vi "TC Max and Min Benchmark.vi"() -> ()   [LabVIEW 2010]
uses:
  <vilib>/eio/EIONode/EIONode.xnode
panel:
  out "Minimum Reached":fxp<+/-,24,-2> format="%.26g"
  out "Maximum Reached":fxp<+/-,24,-2> format="%.26g"
  out "Current TC Signal":fxp<+/-,24,-2> format="%.26g"
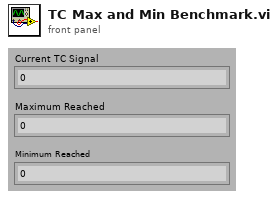
[diagram p1: front panel]
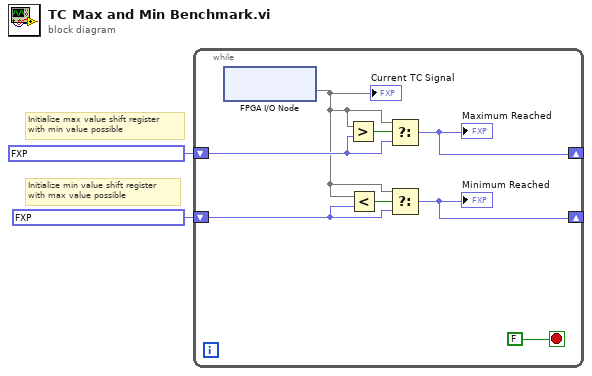
[diagram p0: block diagram]
diagram:
  # "Initialize max value shift register\nwith min value possible"
  # "Initialize min value shift register\nwith max value possible"
  n1 = while {
    shift-right: [w7] -> _
    shift-left: fxp<+/-,24,-2> -0.125 -> [w8]
    shift-right: [w3] -> _
    shift-left: fxp<+/-,24,-2> 0.1249999850988388 -> [w4]
    stop <- FALSE stop-if-true
    n2 = xnode "FPGA I/O Node"() -> ("Mod1/TC0"=w5)  [unwired: 1 in, 1 out]
    "Current TC Signal" <- w5
    n3 = Greater?(x=w5, y=w8) -> (0:w9:bool)
    n4 = Less?(x=w5, y=w4) -> (x < y?=w6:bool)
    n5 = Select(t=w5, s=w9, f=w8) -> (s? t:f=w7:fxp<+/-,24,-2>)
    "Maximum Reached" <- w7
    n6 = Select(t=w5, s=w6, f=w4) -> (s? t:f=w3:fxp<+/-,24,-2>)
    "Minimum Reached" <- w3
  }
